vi "Parse Endpoint.vi"(11 "Module/Endpoint":string) -> (2 "Endpoint":string, 3 "Module":string)   [LabVIEW 2020, in "Routing and Faulting System Explorer.lvlib"]
uses:
  Routing and Faulting System Explorer.lvlib
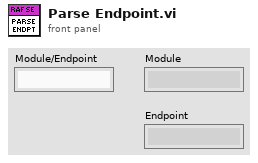
[diagram p1: front panel]
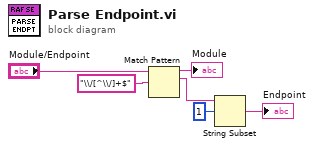
[diagram p0: block diagram]
diagram:
  n1 = Match Pattern(string="Module/Endpoint", regular expression="\\/[^\\/]+$") -> (before substring=→"Module":string, match substring=w3:string)  [unwired: 1 in, 2 out]
  n2 = String Subset(string=w3, offset (0)=1) -> (substring=→"Endpoint":string)  [unwired: 1 in]
